vi "Unpack.vi"(10 "data":variant, 11 "X":dbl[](array[numeric])) -> (1 "Control":dbl[][](array[numeric]), 2 "State":dbl[][](array[numeric]), 3 "Time":dbl[](array[numeric]))   [LabVIEW 2020]
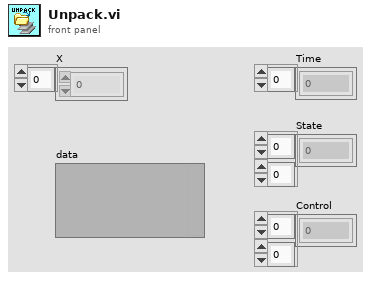
[diagram p1: front panel]
types:
  T1 = cluster{"nGrid":dbl, "nControl":i32, "nState":i32}
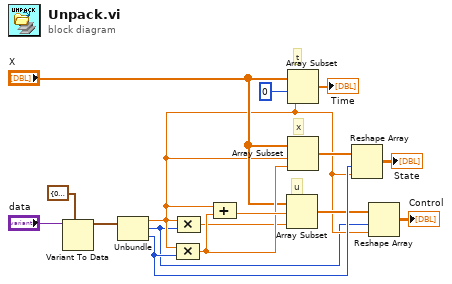
[diagram p0: block diagram]
diagram:
  # "u"
  # "x"
  # "t"
  n1 = Variant To Data(type=T1 {"nGrid"=0.0, "nControl"=0, "nState"=0} ("output cluster"), Variant="data") -> (data=w9:T1)  [unwired: 1 in, 1 out]
  n2 = Unbundle(w9) -> ("nGrid"=w4:dbl, "nControl"=w3:i32, "nState"=w6:i32)
  n3 = Compound Arithmetic op=MULTIPLY(w4, w6) -> (w14:dbl)
  n4 = Compound Arithmetic op=MULTIPLY(w4, w3) -> (w13:dbl)
  n5 = Compound Arithmetic op=ADD(w4, w14) -> (w15:dbl)
  n6 = Array Subset(array="X", index=w15, length=w13) -> (w5:dbl[])
  n7 = Array Subset(array="X", index=0, length=w4) -> (→"Time":dbl[])
  n8 = Array Subset(array="X", index=w4, length=w14) -> (w7:dbl[])
  n9 = Reshape Array(w7, w6, w4) -> (→"State":dbl[][])
  n10 = Reshape Array(w5, w3, w4) -> (→"Control":dbl[][])
